vi "testReadSHWFSdata.vi"(8 "error in (no error)":errorcluster) -> (0 "error out":errorcluster)   [LabVIEW 2016]
doc: "Test to read the SHWFS file."
uses:
  OptStateEsti/OptStateEsti.lvclass
  StrictDef/InstName.ctl
  OfcFunc.lvlib
  <vilib>/addons/_JKI Toolkits/Caraya/classes/Test/Test.lvclass
  <vilib>/addons/_JKI Toolkits/Caraya/classes/Assert/Assert.lvclass
panel:
  in  "OptStateEsti.lvclass":refnum<class "OptStateEsti.lvclass">
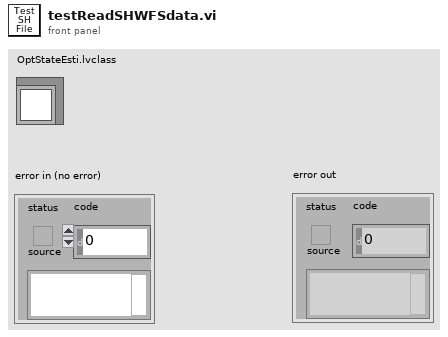
[diagram p1: front panel]
types:
  T1 = typedef "OfcFunc.lvlib/InstName.ctl" = enum16{"lsst", "comcam"}
  T2 = cluster{"Config Dir":path, "Inst Name":T1, "Config File Name":string, "Mapping File Name":string, "Wavelength Table":string, "Intrinc Zk File Name":string, "y2 Corection File Name":string, "Index DOF File Name":string}
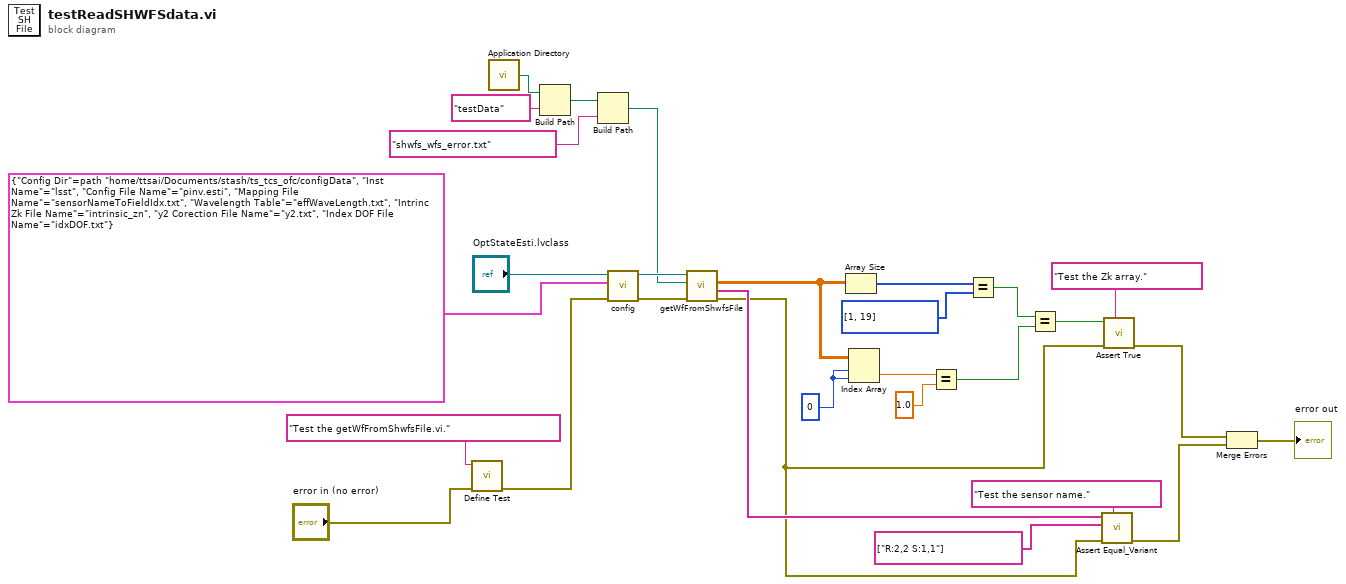
[diagram p0: block diagram]
diagram:
  w14 = 0 ("index (row)")
  n1 = call <vilib>:"Define Test.vi"("error in (no error)"="error in (no error)", "Label (VI Title)"="Test the getWfFromShwfsFile.vi.") -> ("error out"=w26:errorcluster)  [unwired: 9 in]
  n2 = call <vilib>:"Application Directory.vi"() -> ("Application Directory"=w5:path)
  n3 = Build Path(base path=w5, name or relative path="testData") -> (appended path=w3:path)
  n4 = Build Path(base path=w3, name or relative path="shwfs_wfs_error.txt") -> (appended path=w1:path)
  n5 = call "config.vi"("error in (no error)"=w26, "Configuration"=T2 {"Config Dir"=path "/home/ttsai/Documents/stash/ts_tcs_ofc/configData", "Inst Name"=enum."lsst", "Config File Name"="pinv.esti", "Mapping File Name"="sensorNameToFieldIdx.txt", "Wavelength Table"="effWaveLength.txt", "Intrinc Zk File Name"="intrinsic_zn", "y2 Corection File Name"="y2.txt", "Index DOF File Name"="idxDOF.txt"}, "OptStateEsti in"="OptStateEsti.lvclass") -> ("error out"=w23:errorcluster, "OptStateEsti out"=w24:refnum<class "OptStateEsti.lvclass">)  [unwired: 7 in]
  n6 = call "getWfFromShwfsFile.vi"("error in (no error)"=w23, "Wfs Err Data"=w1, "OptStateEsti in"=w24) -> ("error out"=w11:errorcluster, "Sensor Name"=w12:string[], "Wavefront Error"=w22:dbl[][])  [unwired: 5 in, 1 out]
  n7 = Array Size(array=w22) -> (size(s)=w21:i32[])
  n8 = Index Array(array=w22, index (row)=w14, index (col)=w14) -> (element=w19:dbl)
  n9 = Equal?(x=w19, y=1.0) -> (x = y?=w17:bool)
  n10 = Equal?(x=w21, y=i32[] [1, 19]) -> (x = y?=w18:bool)
  n11 = Equal?(x=w18, y=w17) -> (x = y?=w16:bool)
  n12 = call <vilib>:"Assert Equal_Variant.vi"("Label"="Test the sensor name.", "error in (no error)"=w11, "Y"=string[] ["R:2,2 S:1,1"], "X"=w12) -> ("error out"=w9:errorcluster)  [unwired: 7 in]
  n13 = call <vilib>:"Assert True.vi"("Label"="Test the Zk array.", "error in (no error)"=w11, "True?"=w16) -> ("error out"=w10:errorcluster)  [unwired: 8 in]
  n14 = Merge Errors(w10, w9) -> (→"error out":errorcluster)
